vi "Generalized Fourier Spectrum.vi"() -> ()   [LabVIEW 2020]
doc: "Calculates the Fourier and Lomb spectrum for signals evenly spaced or randomly spaced in time."
uses:
  <vilib>/Analysis/2dsp.llb/Power Spectrum (DBL).vi
  <vilib>/gmath/NI_Gmath.lvlib
  <vilib>/Analysis/NI_AALPro.lvlib
panel:
  in  "Tab Control":enum32{"Introduction", "Demonstration"}(tab)
  out "Time Response of mixed signals":cluster{dbl[], dbl[]}(graph)
  in  "Randomly spaced":bool
  out "Fourier and Lomb Spectrum":T1(graph)
  in  "Offset":dbl(slide) scale=0.0..10.0
  in  "Frequency 1":dbl(knob)=4.0 scale=0.0..10.0
  in  "Frequency 2":dbl(knob) scale=0.0..10.0
  in  "Frequency 3":dbl(knob) scale=0.0..20.0
  in  "Frequency 4":dbl(knob) scale=0.0..20.0
  out "Fourier Power":dbl=0.49755803831203815 format="%0.2f"
  out "Lomb Power":dbl=0.49755803831203804 format="%0.2f"
  in  "Stop":bool
  # "Overview: Calculates the Fourier and Lomb spectrum for signals evenly spaced or randomly spaced in time.\nThe Fourier Power Spectrum of a signal X = {x0,x1,...,xn-1} and Xtime = [t0,t1,...,tn-1} can be calculated using the FFT algorithm if the points tj are evenly spaced.\nThis method cannot be used when working with unevenly spaced data points.  In this case the Lomb periodogram yields an approximation of the power spectrum. The Lomb periodogram is defined as follows:"
  # "w is the angular frequency w= 2pf.\nThe VI demonstrates the calculation of the Lomb periodogram for a mix of different frequencies, where the signal is unevenly sampled.\nRequirements: LabVIEW Full Development System\nInstructions: \n1. Run the VI.\n2. Select the Demonstration tab and change the Frequency values. Verify that the results of the Fourier and Lomb Spectrum match each other.\n3. Click the Randomly Spaced button and verify that only the Lomb technique shows the correct spectrum.\n4. Click Stop to stop the VI."
  # "Elementary frequencies are multiples of 1/T, where T=2*pi"
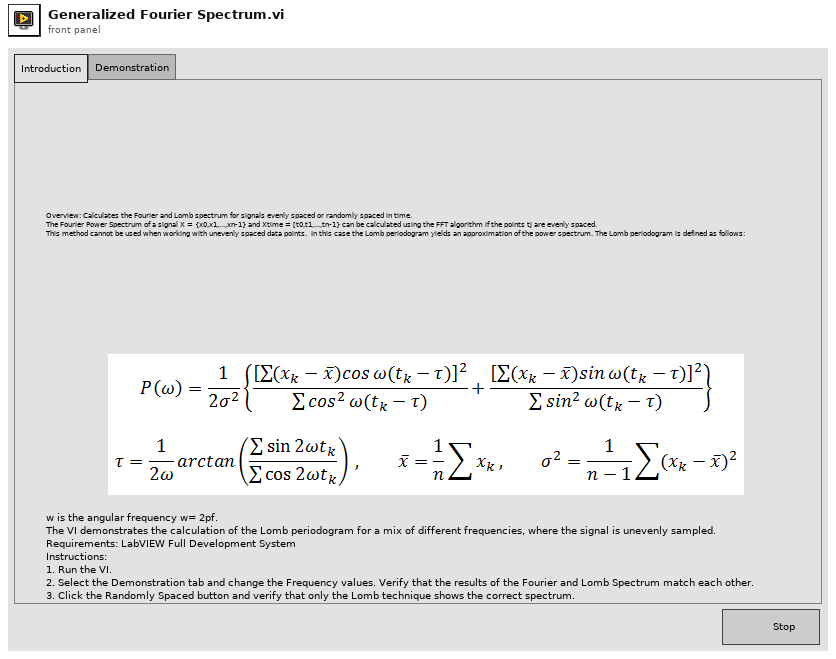
[diagram p1: front panel]
types:
  T1 = cluster{"Power Spectrum FFT {X} Frequency":dbl[], "Power Spectrum FFT {X}":dbl[]}[]
  T2 = cluster{"Power Spectrum FFT {X} Frequency":dbl[], "Power Spectrum FFT {X}":dbl[]}
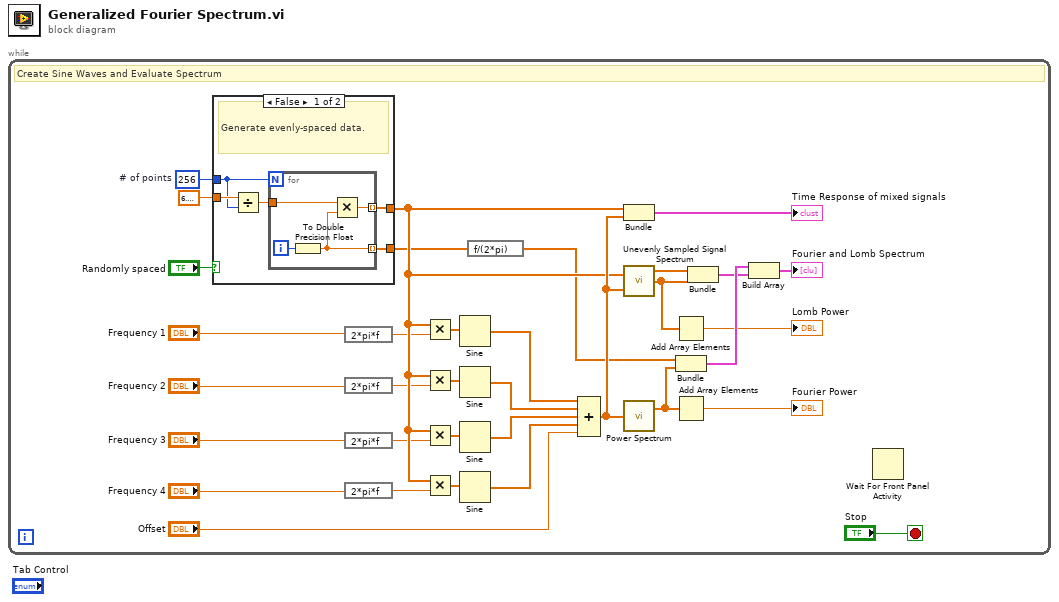
[diagram p0: block diagram]
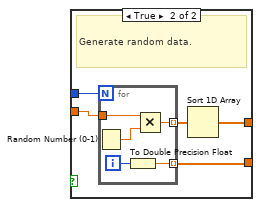
[diagram p2: hidden frame]
diagram:
  n1 = while {
    stop <- "Stop" stop-if-true
    w27 = u32 256  # # of points
    # "Create Sine Waves and Evaluate Spectrum"
    n2 = case shown="False" "Randomly spaced" {
      tunnel: w27 -> [w35 w48]
      tunnel: [w39 w47] -> w7
      tunnel: [w38 w44] -> w23
      tunnel: 6.283185307179586 -> [w37 w45]
      frame False {
        # "Generate evenly-spaced data."
        n3 = Divide(x=w37, y=w35) -> (x/y=w36:dbl)
        n4 = for {
          N: w35 -> [_]
          tunnel: [w40] -> w39 mode=indexing
          tunnel: w36 -> [w43]
          tunnel: [w42] -> w38 mode=indexing
          i -> [w41]
          n5 = To Double Precision Float(number=w41) -> (double precision float=w40:dbl)
          n6 = Multiply(x=w43, y=w40) -> (x*y=w42:dbl)
        }
      }
      frame True {
        # "Generate random data."
        n7 = for {
          N: w48 -> [_]
          tunnel: w45 -> [w53]
          tunnel: [w51] -> w46 mode=indexing
          tunnel: [w49] -> w47 mode=indexing
          i -> [w50]
          n8 = Random Number (0-1)() -> (number: 0 to 1=w52:dbl)
          n9 = To Double Precision Float(number=w50) -> (double precision float=w49:dbl)
          n10 = Multiply(x=w53, y=w52) -> (x*y=w51:dbl)
        }
        n11 = Sort 1D Array(array=w46) -> (sorted array=w44:dbl[])
      }
    }
    n12 = expression code="2*pi*f"("Frequency 1") -> (w9:dbl)
    n13 = expression code="2*pi*f"("Frequency 2") -> (w8:dbl)
    n14 = expression code="2*pi*f"("Frequency 3") -> (w13:dbl)
    n15 = expression code="2*pi*f"("Frequency 4") -> (w14:dbl)
    n16 = Multiply(x=w23, y=w9) -> (x*y=w33:dbl[])
    n17 = Multiply(x=w23, y=w8) -> (x*y=w34:dbl[])
    n18 = Multiply(x=w23, y=w13) -> (x*y=w32:dbl[])
    n19 = Multiply(x=w23, y=w14) -> (x*y=w31:dbl[])
    n20 = Sine(x=w33) -> (sin(x)=w4:dbl[])
    n21 = Sine(x=w34) -> (sin(x)=w5:dbl[])
    n22 = Sine(x=w32) -> (sin(x)=w2:dbl[])
    n23 = Sine(x=w31) -> (sin(x)=w1:dbl[])
    n24 = expression code="f/(2*pi)"(w7) -> (w6:dbl[])
    n25 = Compound Arithmetic op=ADD(w4, w5, w2, w1, "Offset") -> (w24:dbl[])
    n26 = Bundle(w23, w24) -> (→"Time Response of mixed signals":cluster{dbl[], dbl[]})  [unwired: 1 in]
    n27 = call <vilib>:"Unevenly Sampled Signal Spectrum.vi"("XTime"=w23, "X"=w24) -> ("Power Spectrum FFT {X} Frequency"=w29:dbl[], "Power Spectrum FFT {X}"=w21:dbl[])  [unwired: 1 out]
    n28 = call-poly <vilib>:"Power Spectrum.vi"("X"=w24) -> ("Power Spectrum"=w22:dbl[])  [unwired: 1 out]
    n29 = Add Array Elements(numeric array=w21) -> (sum=→"Lomb Power":dbl)
    n30 = Bundle(w6, "Power Spectrum"=w22) -> (w30:cluster{dbl[], "Power Spectrum":dbl[]})  [unwired: 1 in]
    n31 = Add Array Elements(numeric array=w22) -> (sum=→"Fourier Power":dbl)
    n32 = Bundle("Power Spectrum FFT {X} Frequency"=w29, "Power Spectrum FFT {X}"=w21) -> (w28:T2)  [unwired: 1 in]
    n33 = Build Array(w30, w28) -> (→"Fourier and Lomb Spectrum":T1)
    n34 = Wait For Front Panel Activity() -> ()  [unwired: 3 in, 1 out]
  }
